vi "sub_DO-chs.vi"(7 "onoff":bool=TRUE, 8 "error in":errorcluster, 11 "ch":u8) -> (0 "error out":errorcluster)   [LabVIEW 2019]
uses:
  _ctrl/rw.ctl
  cnt_Relay.ctl
  _ctrl/create-rw-close.ctl
  _ctrl/start.ctl
  Durability/common/Global 1.vi
  <vilib>/DAQmx/create/channels.llb/DAQmx Create Channel (DO-Digital Output).vi
  <vilib>/DAQmx/write.llb/DAQmx Write (Digital Bool 1Line 1Point).vi
panel:
  in  "ch-array 2":cluster{"ch":u8, "in-out":bool, "onoff":bool}[](array[cluster])
  out "ch":string
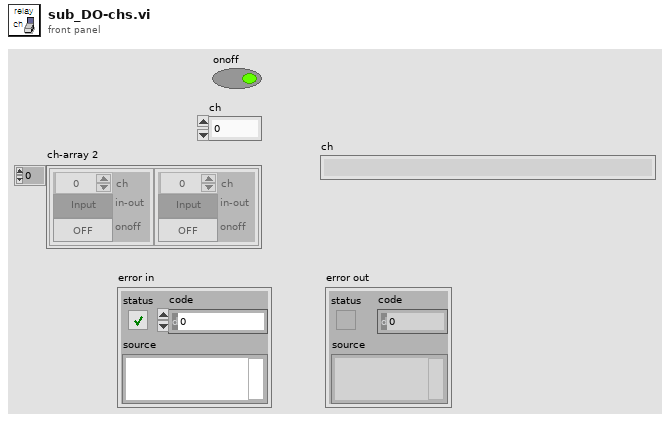
[diagram p1: front panel]
types:
  T1 = typedef "rw.ctl" = enum16{"read", "write"}
  T2 = typedef "cnt_Relay.ctl" = enum32{"R_Load", "R_out1", "R_out2", "R_out3", "R_out4", "R_out5", "R_out6", "R8", "R9", "R10", "R11", "R12", "R13", "R14", "R15", "R16", "R_in1", "R_in2", "R_in3", "R_in4", "R_in5", "R_in6", "R23", "R24", "R25", "R26", "R27", "R_red", "R_yellow", "R_green", "R_buz", "R_purple"}
  T3 = typedef "start.ctl" = enum16{"init", "open", "set", "start", "stop", "read", "read_items", "query", "close", "T_single", "reset", "exit"}
  T4 = typedef "create-rw-close.ctl" = enum16{"create", "write", "read", "delete", "close"}
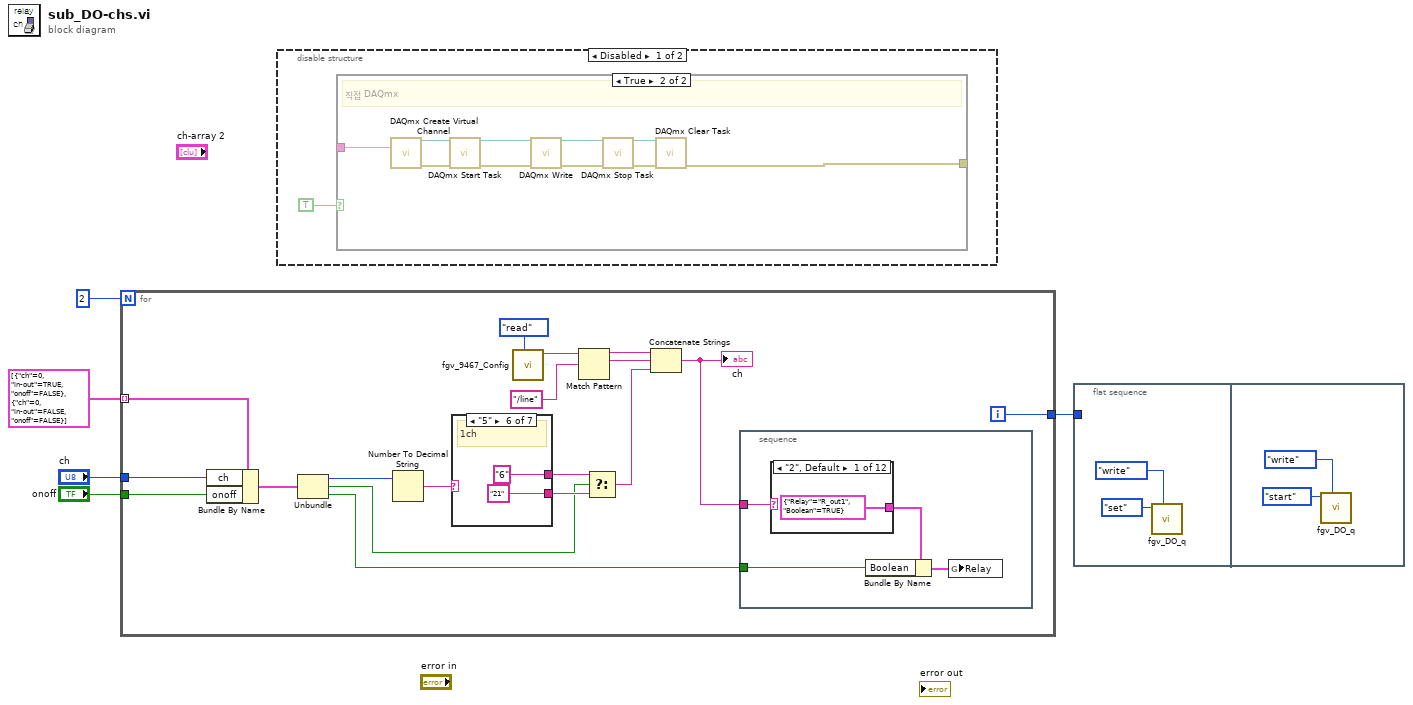
[diagram p0: block diagram]
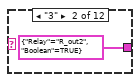
[diagram p4: hidden frame]
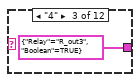
[diagram p5: hidden frame]
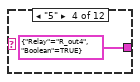
[diagram p6: hidden frame]
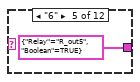
[diagram p7: hidden frame]
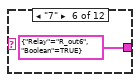
[diagram p8: hidden frame]
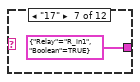
[diagram p9: hidden frame]
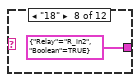
[diagram p10: hidden frame]
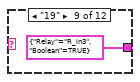
[diagram p11: hidden frame]
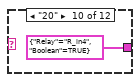
[diagram p12: hidden frame]
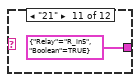
[diagram p13: hidden frame]
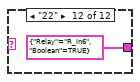
[diagram p14: hidden frame]
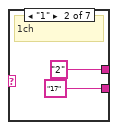
[diagram p16: hidden frame]
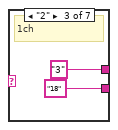
[diagram p17: hidden frame]
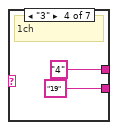
[diagram p18: hidden frame]
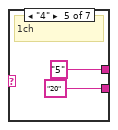
[diagram p19: hidden frame]
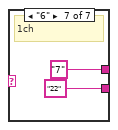
[diagram p20: hidden frame]
diagram:
  n1 = for {
    N: 2 -> [_]
    tunnel: cluster{"ch":u8, "in-out":bool, "onoff":bool}[] [{"ch"=0, "in-out"=TRUE, "onoff"=FALSE}, {"ch"=0, "in-out"=FALSE, "onoff"=FALSE}] ("ch-array") -> [w9] mode=indexing
    tunnel: [w10] -> w5
    tunnel: "ch" -> [w8]
    tunnel: "onoff" -> [w6]
    i -> [w10]
    n2 = Bundle By Name(cluster=w9, "ch"=w8, "onoff"=w6) -> (w7:cluster{"ch":u8, "in-out":bool, "onoff":bool})
    n3 = Unbundle(w7) -> ("ch"=w14:u8, "in-out"=w12:bool, "onoff"=w13:bool)
    n4 = Number To Decimal String(number=w14) -> (decimal integer string=w22:string)  [unwired: 1 in]
    n5 = case shown="\"5\"" w22 {
      tunnel: [_ "17" ("string") "18" ("string") "19" ("string") "20" ("string") "21" ("string") "22" ("string")] -> w17
      tunnel: [_ "2" ("string") "3" ("string") "4" ("string") "5" ("string") "6" ("string") "7" ("string")] -> w16
      frame "False", Default {
      }
      frame "1" {
        # "1ch"
      }
      frame "2" {
        # "1ch"
      }
      frame "3" {
        # "1ch"
      }
      frame "4" {
        # "1ch"
      }
      frame "5" {
        # "1ch"
      }
      frame "6" {
        # "1ch"
      }
    }
    n6 = call "fgv_9467_Config.vi"("cmd"=rw."read") -> ("cDAQ-9467 Config 2"=w21:tag)  [unwired: 10 in]
    n7 = Match Pattern(string=w21, regular expression="/line" ("string")) -> (before substring=w19:string, match substring=w18:string)  [unwired: 1 in, 2 out]
    n8 = Select(t=w16, s=w12, f=w17) -> (s? t:f=w15:string)
    n9 = Concatenate Strings(w19, w18, w15) -> (w11:string)
    "ch" <- w11
    n10 = stacked-sequence {
      tunnel: w11 -> [w27]
      tunnel: w13 -> [w26]
      frame #0 {
        n11 = case shown="\"2\", Default" w27 {
          tunnel: [cluster{"Relay":T2, "Boolean":bool} {"Relay"=enum."R_out1", "Boolean"=TRUE} ("Relay") cluster{"Relay":T2, "Boolean":bool} {"Relay"=enum."R_out2", "Boolean"=TRUE} ("Relay") cluster{"Relay":T2, "Boolean":bool} {"Relay"=enum."R_out3", "Boolean"=TRUE} ("Relay") cluster{"Relay":T2, "Boolean":bool} {"Relay"=enum."R_out4", "Boolean"=TRUE} ("Relay") cluster{"Relay":T2, "Boolean":bool} {"Relay"=enum."R_out5", "Boolean"=TRUE} ("Relay") cluster{"Relay":T2, "Boolean":bool} {"Relay"=enum."R_out6", "Boolean"=TRUE} ("Relay") cluster{"Relay":T2, "Boolean":bool} {"Relay"=enum."R_in1", "Boolean"=TRUE} ("Relay") cluster{"Relay":T2, "Boolean":bool} {"Relay"=enum."R_in2", "Boolean"=TRUE} ("Relay") cluster{"Relay":T2, "Boolean":bool} {"Relay"=enum."R_in3", "Boolean"=TRUE} ("Relay") cluster{"Relay":T2, "Boolean":bool} {"Relay"=enum."R_in4", "Boolean"=TRUE} ("Relay") cluster{"Relay":T2, "Boolean":bool} {"Relay"=enum."R_in5", "Boolean"=TRUE} ("Relay") cluster{"Relay":T2, "Boolean":bool} {"Relay"=enum."R_in6", "Boolean"=TRUE} ("Relay")] -> w24
          frame "2", Default {
          }
          frame "3" {
          }
          frame "4" {
          }
          frame "5" {
          }
          frame "6" {
          }
          frame "7" {
          }
          frame "17" {
          }
          frame "18" {
          }
          frame "19" {
          }
          frame "20" {
          }
          frame "21" {
          }
          frame "22" {
          }
        }
        n12 = Bundle By Name(cluster=w24, "Boolean"=w26) -> (w25:cluster{"Relay":T2, "Boolean":bool})
        n13 = global write "Global 1.vi" "Relay"(w25) -> ()
      }
    }
  }
  n14 = disable-structure shown="Disabled" {
    frame Disabled {
      n15 = case shown="True" TRUE {
        tunnel: _ -> [_ w54]
        tunnel: [_ w53] -> _
        frame False {
          # "매인 생상/소비"
        }
        frame True {
          # "직접 DAQmx"
          n16 = call-poly <vilib>:"DAQmx Create Virtual Channel.vi"("lines"=w54) -> ("task out"=w61:refnum<k21>, "error out"=w62:errorcluster)  [unwired: 13 in]
          n17 = call <vilib>:"DAQmx Start Task.vi"("task/channels in"=w61, "error in"=w62) -> ("task out"=w58:refnum<k21>, "error out"=w57:errorcluster)  [unwired: 12 in]
          n18 = call-poly <vilib>:"DAQmx Write.vi"("task/channels in"=w58, "error in"=w57) -> ("task out"=w56:refnum<k21>, "data"=w63:bool, "error out"=w55:errorcluster)  [unwired: 10 in, 1 out]
          n19 = call <vilib>:"DAQmx Stop Task.vi"("task/channels in"=w56, "error in"=w55) -> ("task out"=w60:refnum<k21>, "error out"=w59:errorcluster)  [unwired: 12 in]
          n20 = call <vilib>:"DAQmx Clear Task.vi"("task in"=w60, "error in"=w59) -> ("error out"=w53:errorcluster)  [unwired: 13 in]
        }
      }
    }
    frame Enabled {
    }
  }
  n21 = flat-sequence {
    tunnel: w5 -> [_]
    frame #0 {
      n22 = call "fgv_DO_q.vi"("cmd"=create-rw-close."write", "data"=start."set") -> ()  [unwired: 8 in, 2 out]
    }
    frame #1 {
      n23 = call "fgv_DO_q.vi"("cmd"=create-rw-close."write", "data"=start."start") -> ()  [unwired: 8 in, 2 out]
    }
  }
